vi "XNET UDP Socket Read (Text).vi"(8 "error in":errorcluster, 9 "timeout ms (25000)":i32=25000, 10 "max size (548)":i32=548, 11 "socket in":refnum<k20>) -> (0 "error out":errorcluster, 2 "data":string, 3 "socket out":refnum<k20>, 4 "remote port":u16, 6 "remote address":string)   [LabVIEW 2018]
doc: "Reads a string datagram from a UDP socket."
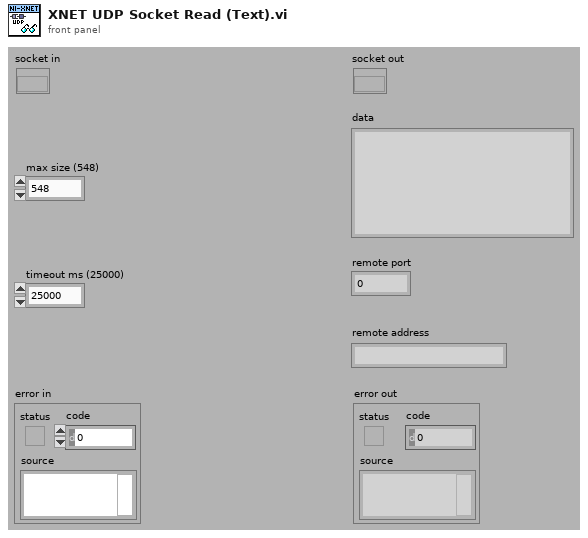
[diagram p1: front panel]
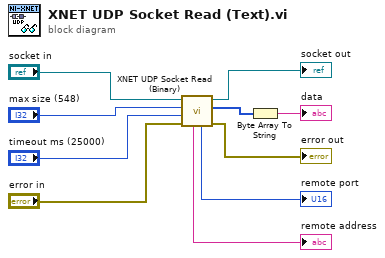
[diagram p0: block diagram]
diagram:
  n1 = call "XNET UDP Socket Read (Binary).vi"("error in"="error in", "timeout ms (25000)"="timeout ms (25000)", "max size (548)"="max size (548)", "socket in"="socket in") -> ("error out"=→"error out":errorcluster, "data"=w2:u8[], "socket out"=→"socket out":refnum<k20>, "remote port"=→"remote port":u16, "remote address"=→"remote address":string)  [unwired: 3 in]
  n2 = Byte Array To String(unsigned byte array=w2) -> (string=→"data":string)
